vi "CRYSort Time FFT.vi"(9 "Infor":T1, 10 "Fs":dbl=44100.0 min=1.0, 11 "Signal":dbl[](array[numeric])) -> (0 "Amp Spectrum Mag":dbl[][](array[numeric]), 1 "df":dbl format="%.2f", 2 "theta":dbl[](array[numeric]), 3 "r":dbl[](array[numeric]))   [LabVIEW 2013]
uses:
  <vilib>/Analysis/NI_AALPro.lvlib
panel:
  out "Waveform Graph":dbl[](graph)
  # "Short Time FFT"
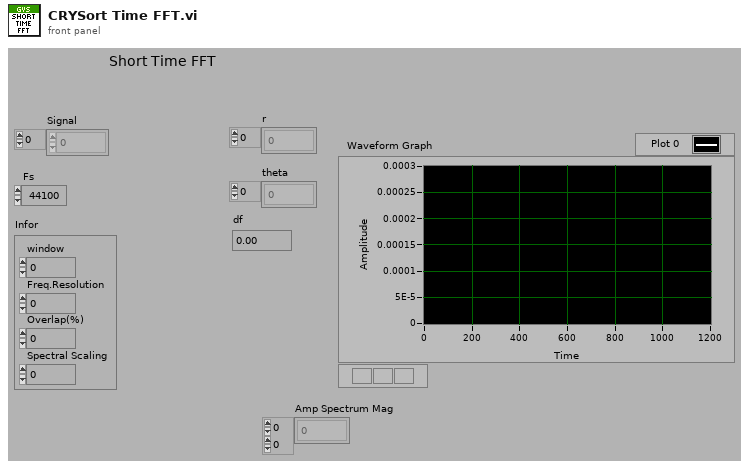
[diagram p1: front panel]
types:
  T1 = cluster{"window":u16, "Freq.Resolution":dbl, "Overlap(%)":dbl, "Spectral Scaling":u16}
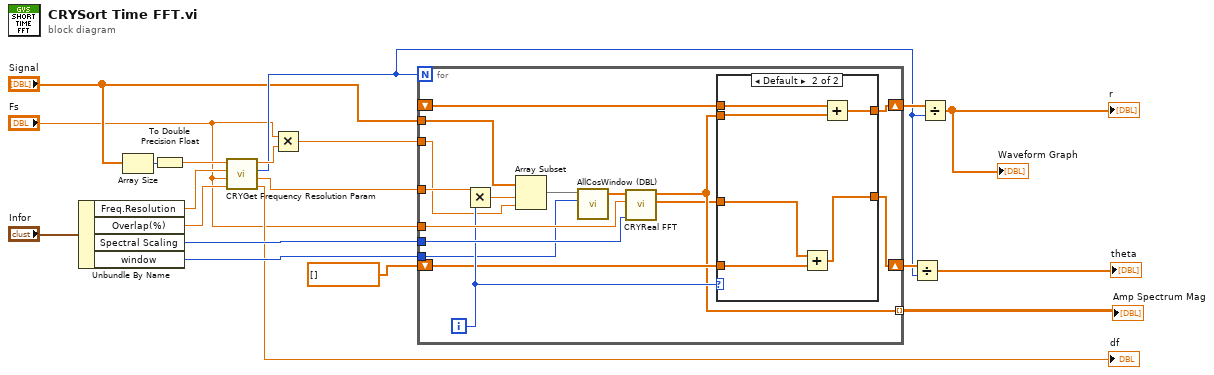
[diagram p0: block diagram]
diagram:
  n1 = Unbundle By Name("Infor") -> ("Freq.Resolution"=w13:dbl, "Overlap(%)"=w19:dbl, "Spectral Scaling"=w15:u16, "window"=w16:u16)
  n2 = Array Size(array="Signal") -> (size(s)=w11:i32)
  n3 = To Double Precision Float(number=w11) -> (double precision float=w10:dbl)
  n4 = call "CRYGet Frequency Resolution Param.vi"("Overlap(%)"=w19, "Fs"="Fs", "Freq Resolution(Hz)"=w13, "Samples"=w10) -> ("Out Freq Resolution(Hz)"=→"df":dbl, "Shift Samples"=w4:dbl, "No. of FFT"=w7:i32, "Record Length(s)"=w18:dbl)  [unwired: 4 in]
  n5 = Multiply(x="Fs", y=w18) -> (x*y=w17:dbl)
  n6 = for {
    N: w7 -> [_]
    tunnel: "Signal" -> [w28]
    tunnel: w4 -> [w36]
    tunnel: w15 -> [w33]
    tunnel: w16 -> [w24]
    tunnel: w17 -> [w29]
    tunnel: "Fs" -> [w34]
    shift-right: [w32] -> w14
    shift-left: _ -> [w31]
    shift-right: [w27] -> w8
    shift-left: dbl[] [] -> [w26]
    tunnel: [w22] -> w2 mode=indexing
    i -> [w30]
    n7 = Multiply(x=w36, y=w30) -> (x*y=w35:dbl)
    n8 = Array Subset(array=w28, index=w35, length=w29) -> (w23:dbl[])
    n9 = call <vilib>:"AllCosWindow (DBL).vi"("window"=w24, "X"=w23) -> ("Windowed X"=w25:dbl[])  [unwired: 1 in, 3 out]
    n10 = call "CRYReal FFT.vi"("Spectral Scaling"=w33, "Fs"=w34, "Signal (V)"=w25) -> ("Amp Spectrum Phase (radians)"=w21:dbl[], "Amp Spectrum Mag"=w22:dbl[])  [unwired: 6 in, 1 out]
    n11 = case shown="Default" w30 {
      tunnel: w22 -> [w38 w39]
      tunnel: [w38 w43] -> w32
      tunnel: w31 -> [_ w44]
      tunnel: w21 -> [w37 w40]
      tunnel: [w37 w41] -> w27
      tunnel: w26 -> [_ w42]
      frame 0 {
      }
      frame Default {
        n12 = Add(x=w40, y=w42) -> (x+y=w41:dbl[])
        n13 = Add(x=w44, y=w39) -> (x+y=w43:dbl[])
      }
    }
  }
  "Amp Spectrum Mag" <- w2
  n14 = Divide(x=w8, y=w7) -> (x/y=→"theta":dbl[])
  n15 = Divide(x=w14, y=w7) -> (x/y=→"r" →"Waveform Graph":dbl[])
